vi "Blob Create.vi"(8 "error in":errorcluster) -> (0 "error out":errorcluster, 3 "Blob":refnum<class "Blob.lvclass">)   [LabVIEW 2020, in "OpenLvVision_OpenCv.lvlib" / "Blob.lvclass"]
doc: "Object by reference!\nDefault constructor."
uses:
  Blob.lvclass
  C:/Users/lukas/Downloads/OpenLvVision_OpenCv/SourceCode/LabView/OpenLvVision_OpenCv/_LvHelpers/EdvrObject/EdvrObject.lvclass
  _LvHelpers/EdvrObject/TypeDef/Edvr.ctl
  _LvHelpers/EdvrObject/EdvrObject.lvclass/EdvrObject.ctl
  _LvHelpers/EdvrObject/EdvrObject.lvclass
  OpenLvVision_OpenCv.lvlib
  Dlls/OlvOpenCvWrapper.dll
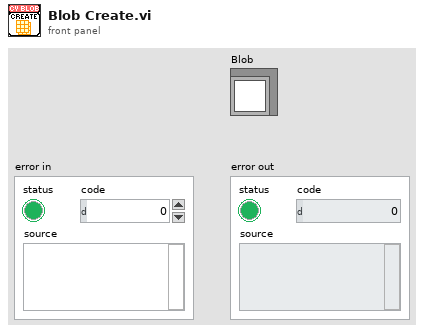
[diagram p1: front panel]
types:
  T1 = typedef "OpenLvVision_OpenCv.lvlib/EdvrObject.lvclass/Edvr.ctl" = refnum<data-value>
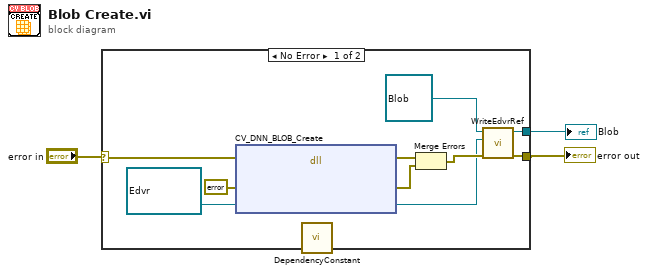
[diagram p0: block diagram]
diagram:
  n1 = case shown="No Error" "error in" {
    selector: "error in" -> [w6 w14]
    tunnel: [w13 w14] -> w2
    tunnel: [w12 _] -> w1
    frame No Error {
      n2 = dll-call lib="C:/Users/lukas/Downloads/OpenLvVision_OpenCv/SourceCode/LabView/OpenLvVision_OpenCv/Dlls/OlvOpenCvWrapper.dll" fn="CV_DNN_BLOB_Create"(error in=w6, "Error"=errorcluster {"status"=FALSE, "code"=0, "source"=""} ("error out"), "edvrRef"=T1 refnum ("Edvr")) -> (error out=w10:errorcluster, "Error"=w9:errorcluster, "edvrRef"=w5:T1)  [unwired: 3 in, 1 out]
      n3 = call "DependencyConstant.vi"() -> ()  [unwired: 12 in]
      n4 = Merge Errors(w10, w9) -> (w7:errorcluster)
      n5 = call "WriteEdvrRef.vi"("error in (no error)"=w7, "Edvr"=w5, "EdvrObject in"=refnum<class "Blob.lvclass"> refnum ("OpenLvVision_OpenCv.lvlib:Blob")) -> ("error out"=w13:errorcluster, "EdvrObject out"=w12:refnum<class "Blob.lvclass">)  [unwired: 7 in]
    }
    frame Error {
    }
  }
  "Blob" <- w1
  "error out" <- w2
